vi "Format Property List.vi"(1 "property names":string[](array[string]), 2 "property values":variant[](array[variant])) -> (0 "strings":string[][](array[string]))   [LabVIEW 2020, in "NI_TDMS File Viewer.lvlib"]
uses:
  <vilib>/Utility/TDMS File Viewer/NI_TDMS File Viewer.lvlib
  <vilib>/Utility/TDMS File Viewer/Global VI for Localized Text.vi
  <vilib>/Utility/Data Type/NI_Data Type.lvlib
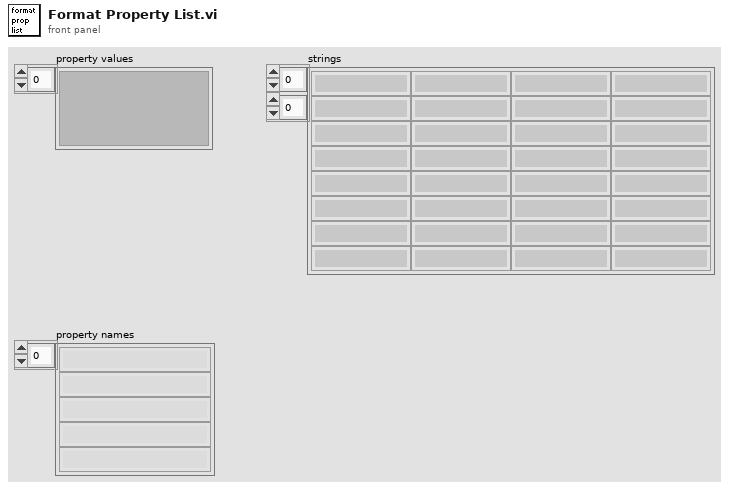
[diagram p1: front panel]
types:
  T1 = typedef "NI_Data Type.lvlib/Data Type.ctl" = enum8{"Invalid Type", "Void", "I8", "I16", "I32", "I64", "U8", "U16", "U32", "U64", "Single Float", "Double Float", "Extended Float", "Single Complex", "Double Complex", "Extended Complex", "Enum U8", "Enum U16", "Enum U32", "Enum U64", "Single Float With Unit", "Double Float With Unit", "Extended Float With Unit", "Single Complex with Unit", "Double Complex with Unit", "Extended Complex with Unit", "Boolean", "String", "Path", "Picture", "Tag", "Array", "Cluster", "Variant", "LV Variant", "Waveform", "Timestamp", "Digital Waveform", "Digital Data", "ExpressData", "Refnum", "External Data", "VI", "Poly VI", "LabVIEW Class Instance", "Fixed Point", "Set Collection", "Map Collection"}
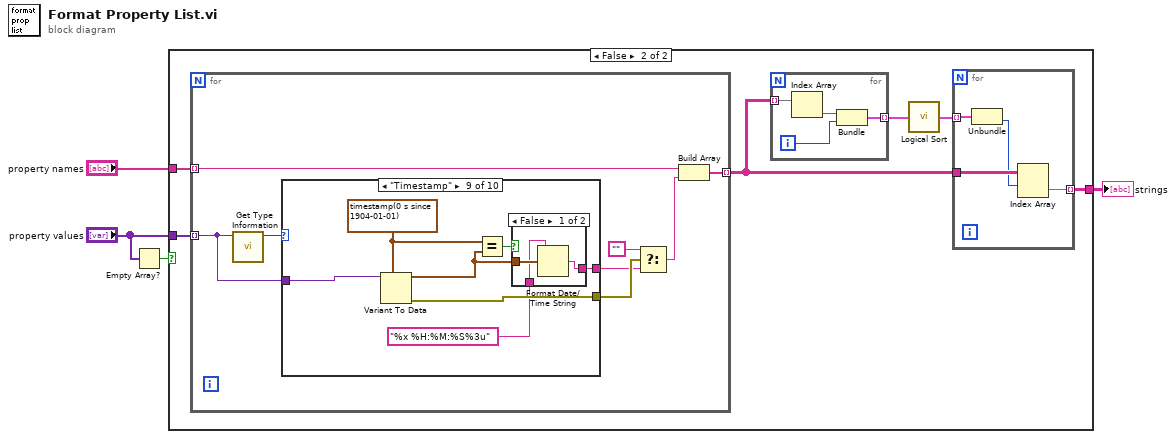
[diagram p0: block diagram]
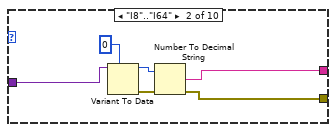
[diagram p4: hidden frame]
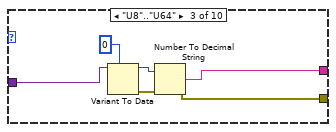
[diagram p5: hidden frame]
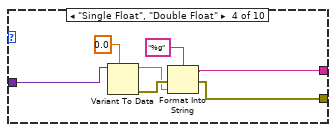
[diagram p6: hidden frame]
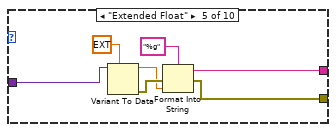
[diagram p7: hidden frame]
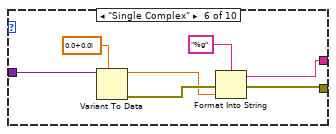
[diagram p8: hidden frame]
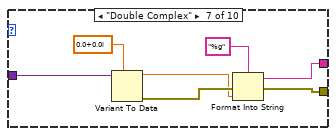
[diagram p9: hidden frame]
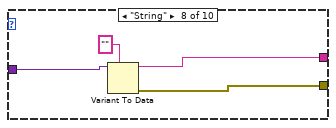
[diagram p10: hidden frame]
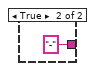
[diagram p11: hidden frame]
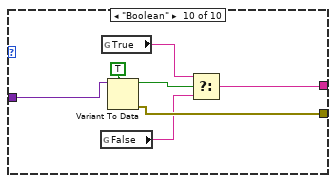
[diagram p12: hidden frame]
diagram:
  n1 = Empty Array?(array="property values") -> (empty?=w2:bool)
  n2 = case shown="False" w2 {
    tunnel: "property names" -> [_ w10]
    tunnel: "property values" -> [_ w9]
    tunnel: [_ w7] -> w1
    frame True {
    }
    frame False {
      n3 = for {
        tunnel: w9 -> [w17] mode=indexing
        tunnel: w10 -> [w16] mode=indexing
        tunnel: [w11] -> w5 mode=indexing
        n4 = call <vilib>:"Get Type Information.vi"("variant"=w17) -> ("type"=w15:T1)  [unwired: 6 in, 4 out]
        n5 = case shown="\"Timestamp\"" w15 {
          tunnel: w17 -> [_ w22 w27 w33 w40 w47 w54 w59 w66 w77]
          tunnel: [_ w23 w28 w34 w41 w48 w55 w60 w67 w78] -> w18
          tunnel: [_ w19 w24 w31 w37 w45 w52 w57 w65 w74] -> w14
          frame Default {
          }
          frame "I8".."I64" {
            n6 = Variant To Data(type=i64 0 ("offset (0)"), Variant=w22) -> (data=w20:i64, error out=w23:errorcluster)  [unwired: 1 in]
            n7 = Number To Decimal String(number=w20) -> (decimal integer string=w19:string)  [unwired: 1 in]
          }
          frame "U8".."U64" {
            n8 = Variant To Data(type=u64 0 ("offset (0)"), Variant=w27) -> (data=w25:u64, error out=w28:errorcluster)  [unwired: 1 in]
            n9 = Number To Decimal String(number=w25) -> (decimal integer string=w24:string)  [unwired: 1 in]
          }
          frame "Single Float", "Double Float" {
            n10 = Variant To Data(type=0.0 ("offset (0)"), Variant=w33) -> (data=w29:dbl, error out=w35:errorcluster)  [unwired: 1 in]
            n11 = Format Into String(format string="%g", error in=w35, w29) -> (resulting string=w31:string, error out=w34:errorcluster)  [unwired: 1 in]
          }
          frame "Extended Float" {
            n12 = Variant To Data(type=ext 0.0 ("offset (0)"), Variant=w40) -> (data=w36:ext, error out=w42:errorcluster)  [unwired: 1 in]
            n13 = Format Into String(format string="%g", error in=w42, w36) -> (resulting string=w37:string, error out=w41:errorcluster)  [unwired: 1 in]
          }
          frame "Single Complex" {
            n14 = Variant To Data(type=csg 0.0+0.0i, Variant=w47) -> (data=w44:csg, error out=w49:errorcluster)  [unwired: 1 in]
            n15 = Format Into String(format string="%g", error in=w49, w44) -> (resulting string=w45:string, error out=w48:errorcluster)  [unwired: 1 in]
          }
          frame "Double Complex" {
            n16 = Variant To Data(type=cdb 0.0+0.0i, Variant=w54) -> (data=w51:cdb, error out=w56:errorcluster)  [unwired: 1 in]
            n17 = Format Into String(format string="%g", error in=w56, w51) -> (resulting string=w52:string, error out=w55:errorcluster)  [unwired: 1 in]
          }
          frame "String" {
            n18 = Variant To Data(type="" ("offset (0)"), Variant=w59) -> (data=w57:string, error out=w60:errorcluster)  [unwired: 1 in]
          }
          frame "Timestamp" {
            w64 = timestamp(0 s since 1904-01-01) ("offset (0)")
            n19 = Variant To Data(type=w64, Variant=w66) -> (data=w63:timestamp, error out=w67:errorcluster)  [unwired: 1 in]
            n20 = Equal?(x=w64, y=w63) -> (x = y?=w62:bool)
            n21 = case shown="False" w62 {
              tunnel: w63 -> [w70 _]
              tunnel: [w69 "-" ("date/time string")] -> w65
              tunnel: "%x %H:%M:%S%3u" ("time format string (%c)") -> [w68 _]
              frame False {
                n22 = Format Date/Time String(time format string (%c)=w68, seconds (now)=w70) -> (date/time string=w69:string)  [unwired: 1 in]
              }
              frame True {
              }
            }
          }
          frame "Boolean" {
            n23 = global read "Global VI for Localized Text.vi" "False"() -> (w73:string)
            n24 = global read "Global VI for Localized Text.vi" "True"() -> (w72:string)
            n25 = Variant To Data(type=TRUE, Variant=w77) -> (data=w75:bool, error out=w78:errorcluster)  [unwired: 1 in]
            n26 = Select(t=w72, s=w75, f=w73) -> (s? t:f=w74:string)
          }
        }
        n27 = Select(t="", s=w18, f=w14) -> (s? t:f=w12:string)
        n28 = Build Array(w16, w12) -> (w11:string[])
      }
      n29 = for {
        tunnel: w5 -> [w82] mode=indexing
        tunnel: [w79] -> w6 mode=indexing
        i -> [w80]
        n30 = Index Array(array=w82) -> (element=w81:string)  [unwired: 1 in]
        n31 = Bundle("False"=w81, w80) -> (w79:cluster{"False":string, i32})  [unwired: 1 in]
      }
      n32 = call <vilib>:"Logical Sort.vi"("Input Array"=w6) -> ("Sorted Array"=w8:cluster{"date/time string":string, i32}[])  [unwired: 8 in]
      n33 = for {
        tunnel: w8 -> [w85] mode=indexing
        tunnel: w5 -> [w86]
        tunnel: [w83] -> w7 mode=indexing
        n34 = Unbundle(w85) -> (w84:i32)  [unwired: 1 out]
        n35 = Index Array(array=w86, index (row)=w84) -> (element=w83:string[])  [unwired: 1 in]
      }
    }
  }
  "strings" <- w1
